vi "TablaPonderacionesACZ.vi"(10 "Tabla Referencia Acústica Generador Externo":string[][](table), 11 "PonderacionesACZ":string[][](array[string])) -> (3 "TablaPonderaciones":string[][](array[string]))   [LabVIEW 2019, in "Base de Datos.lvclass"]
uses:
  Base de Datos.lvclass
panel:
  out "Z":dbl[](array[numeric])
  out "C":dbl[](array[numeric])
  out "A":dbl[](array[numeric])
  out "114dB":dbl[](array[numeric])
  out "94dB":dbl[](array[numeric])
  out "RefAcuGenExt":dbl[][](array[numeric])
  out "Ponderaciones":dbl[][](array[numeric])
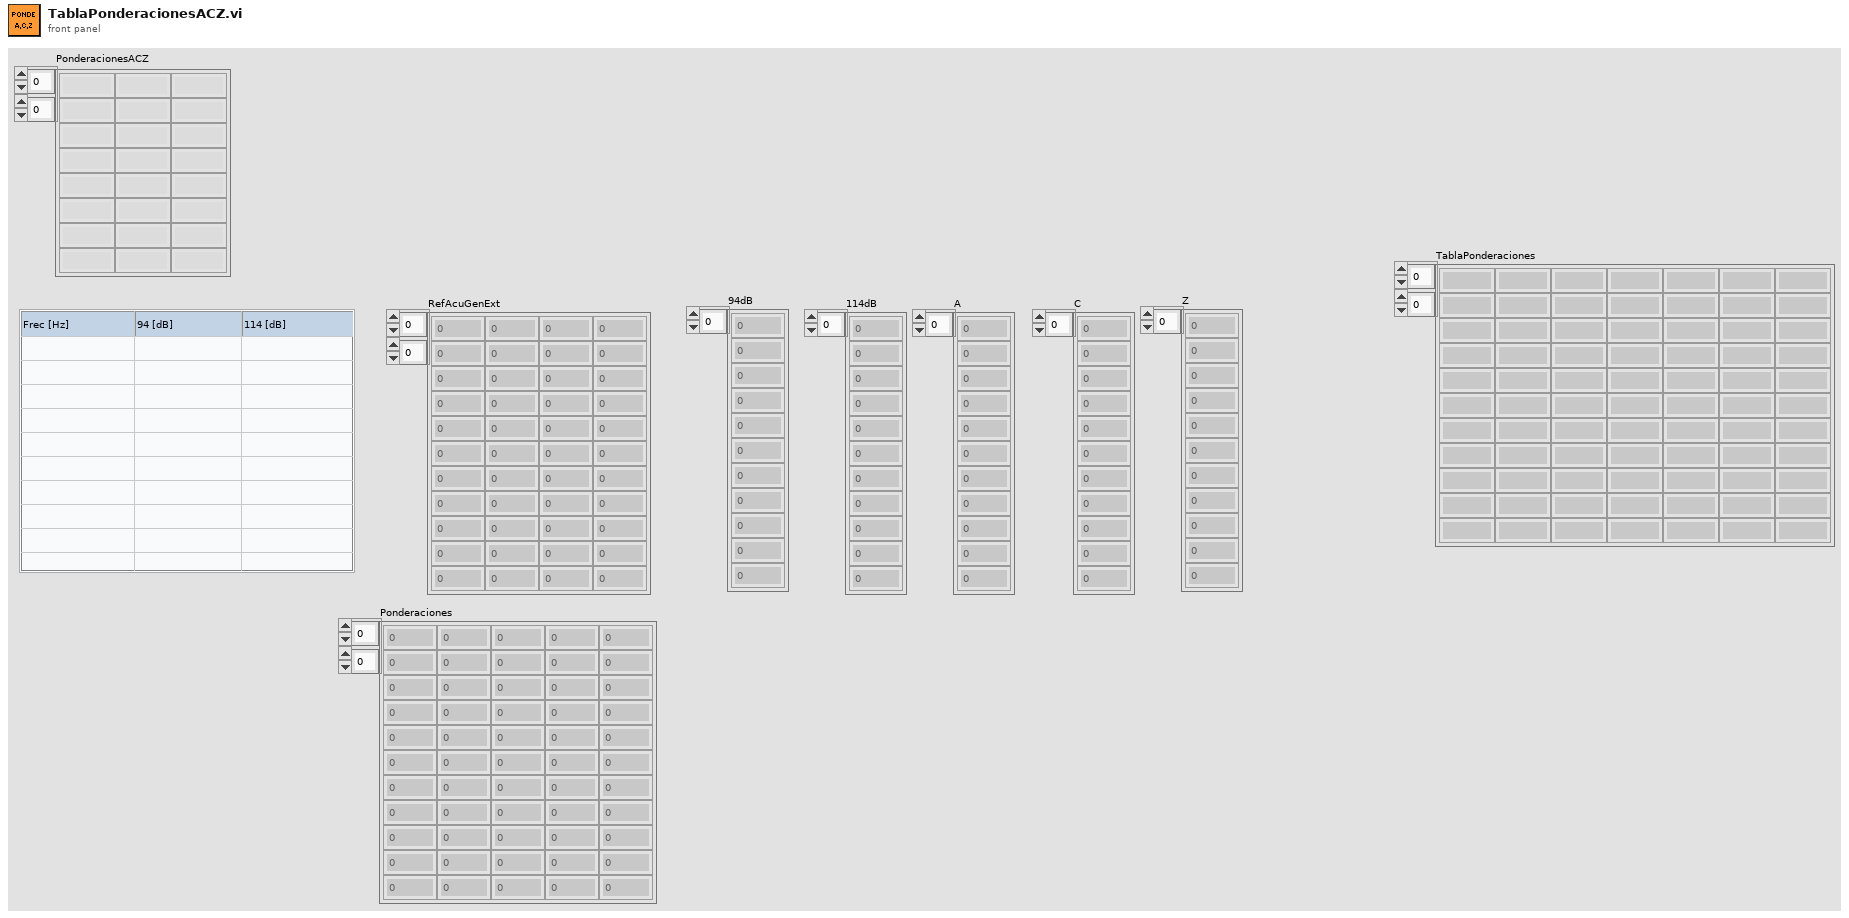
[diagram p1: front panel]
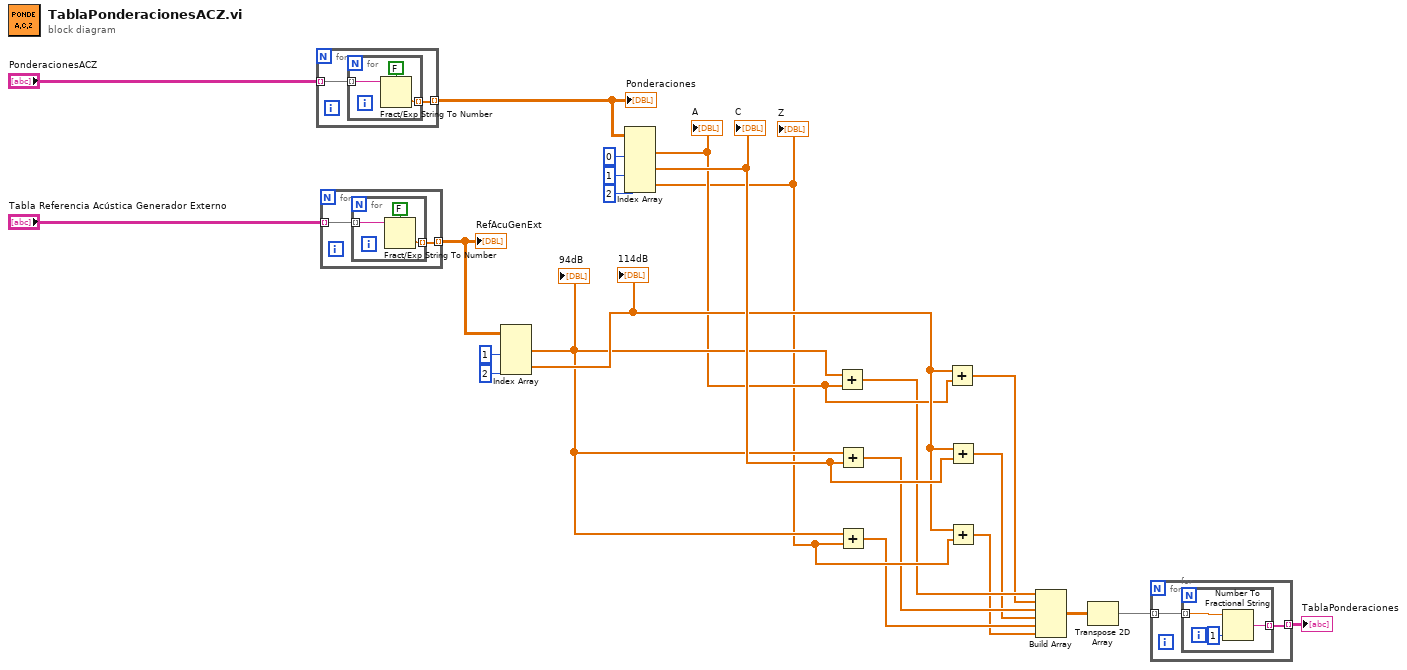
[diagram p0: block diagram]
diagram:
  n1 = for {
    tunnel: "PonderacionesACZ" -> [w25] mode=indexing
    tunnel: [w24] -> w16 mode=indexing
    n2 = for {
      tunnel: w25 -> [w27] mode=indexing
      tunnel: [w26] -> w24 mode=indexing
      n3 = Fract/Exp String To Number(use system decimal point (T)=FALSE, string=w27) -> (number=w26:dbl)  [unwired: 2 in, 1 out]
    }
  }
  "Ponderaciones" <- w16
  n4 = for {
    tunnel: "Tabla Referencia Acústica Generador Externo" -> [w30] mode=indexing
    tunnel: [w29] -> w22 mode=indexing
    n5 = for {
      tunnel: w30 -> [w32] mode=indexing
      tunnel: [w31] -> w29 mode=indexing
      n6 = Fract/Exp String To Number(use system decimal point (T)=FALSE, string=w32) -> (number=w31:dbl)  [unwired: 2 in, 1 out]
    }
  }
  "RefAcuGenExt" <- w22
  n7 = Index Array(array=w22, index (col) #1=1 ("disabled index (col)"), index (col) #2=2 ("index (col)")) -> (element #1=w13:dbl[], element #2=w14:dbl[])  [unwired: 2 in]
  "94dB" <- w13
  "114dB" <- w14
  n8 = Index Array(array=w16, index (col) #1=0 ("disabled index (col)"), index (col) #2=1 ("index (col)"), index (col) #3=2 ("index (col)")) -> (element #1=w12:dbl[], element #2=w15:dbl[], element #3=w11:dbl[])  [unwired: 3 in]
  "A" <- w12
  "C" <- w15
  "Z" <- w11
  n9 = Add(x=w13, y=w12) -> (x+y=w10:dbl[])
  n10 = Add(x=w13, y=w15) -> (x+y=w8:dbl[])
  n11 = Add(x=w13, y=w11) -> (x+y=w6:dbl[])
  n12 = Add(x=w14, y=w12) -> (x+y=w9:dbl[])
  n13 = Add(x=w14, y=w15) -> (x+y=w7:dbl[])
  n14 = Add(x=w14, y=w11) -> (x+y=w5:dbl[])
  n15 = Build Array(w10, w9, w8, w7, w6, w5) -> (w4:dbl[][])
  n16 = Transpose 2D Array(2D array=w4) -> (transposed array=w3:dbl[][])
  n17 = for {
    tunnel: w3 -> [w35] mode=indexing
    tunnel: [w34] -> w2 mode=indexing
    n18 = for {
      tunnel: w35 -> [w38] mode=indexing
      tunnel: [w37] -> w34 mode=indexing
      n19 = Number To Fractional String(number=w38, precision (6)=i16 1) -> (F-format string=w37:string)  [unwired: 2 in]
    }
  }
  "TablaPonderaciones" <- w2
